vi "GDS1104B.vi"() -> ()   [LabVIEW 2014]
panel:
  out "number":u32
  out "read buffer 3":string
  out "read buffer 2":string
  out "before substring":string
  out "after substring":string
  out "Waveform Graph":cluster{dbl, dbl, dbl[]}(graph)
  out "Total Waveform Length":i32
  out "Waveform Start Time":dbl
  out "read buffer":string
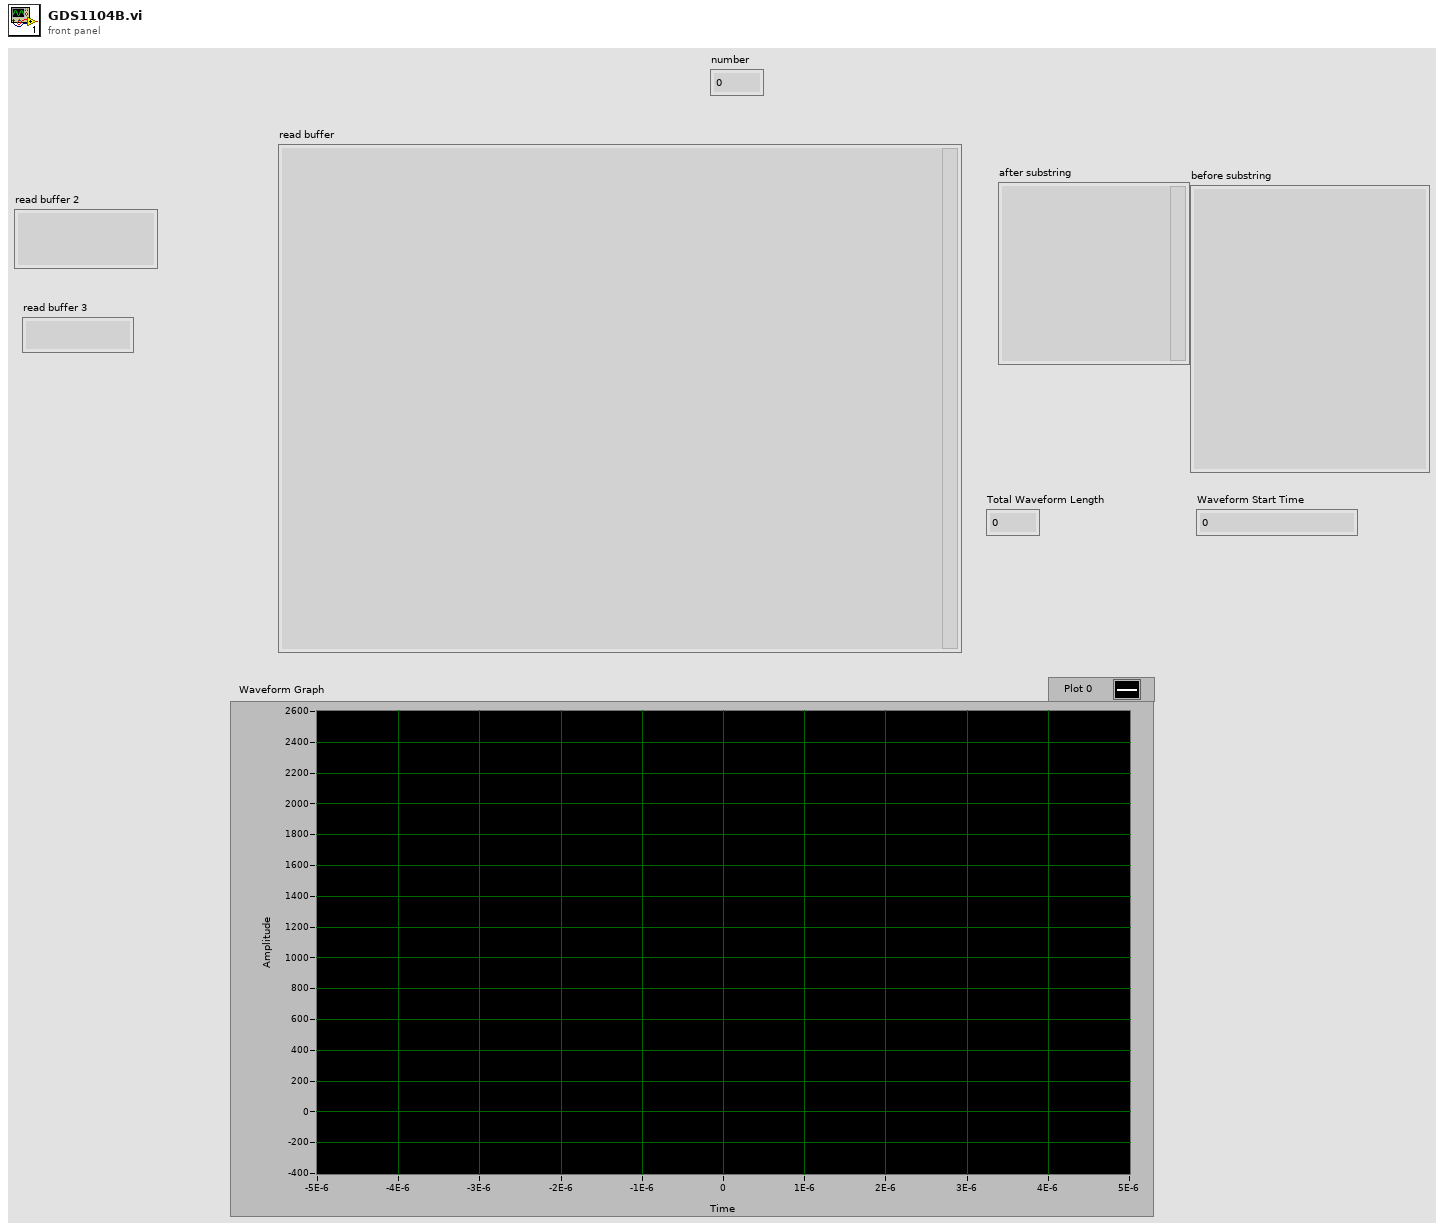
[diagram p1: front panel]
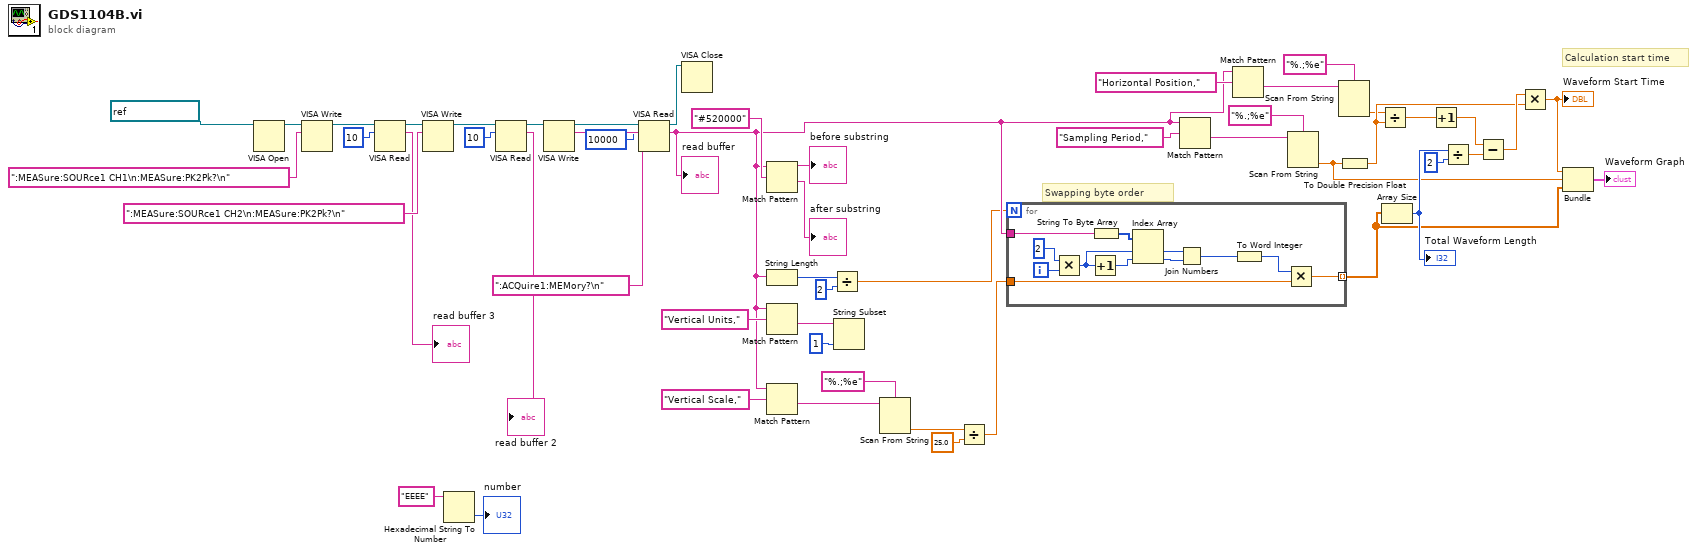
[diagram p0: block diagram]
diagram:
  # "Calculation start time"
  # "Swapping byte order"
  n1 = VISA Open(VISA resource name=refnum<visa-resource-name> "GDS1104B") -> (VISA resource name=w5:refnum<visa-resource-name>)  [unwired: 4 in, 1 out]
  n2 = VISA Write(VISA resource name=w5, write buffer=":MEASure:SOURce1 CH1\n:MEASure:PK2Pk?\n") -> (VISA resource name out=w11:refnum<visa-resource-name>)  [unwired: 1 in, 2 out]
  n3 = VISA Read(VISA resource name=w11, byte count=u32 10) -> (VISA resource name out=w9:refnum<visa-resource-name>, read buffer=→"read buffer 3":string)  [unwired: 1 in, 2 out]
  n4 = VISA Write(VISA resource name=w9, write buffer=":MEASure:SOURce1 CH2\n:MEASure:PK2Pk?\n") -> (VISA resource name out=w15:refnum<visa-resource-name>)  [unwired: 1 in, 2 out]
  n5 = Hexadecimal String To Number(string="EEEE") -> (number=→"number":u32)  [unwired: 2 in, 1 out]
  n6 = VISA Read(VISA resource name=w15, byte count=u32 10) -> (VISA resource name out=w6:refnum<visa-resource-name>, read buffer=→"read buffer 2":string)  [unwired: 1 in, 2 out]
  n7 = VISA Write(VISA resource name=w6, write buffer=":ACQuire1:MEMory?\n") -> (VISA resource name out=w4:refnum<visa-resource-name>)  [unwired: 1 in, 2 out]
  n8 = VISA Read(VISA resource name=w4, byte count=u32 10000) -> (VISA resource name out=w14:refnum<visa-resource-name>, read buffer=w23:string)  [unwired: 1 in, 2 out]
  "read buffer" <- w23
  n9 = VISA Close(VISA resource name=w14) -> ()  [unwired: 1 in, 1 out]
  n10 = Match Pattern(string=w23, regular expression="#520000") -> (before substring=→"before substring":string, after substring=→"after substring":string)  [unwired: 1 in, 2 out]
  n11 = String Length(string=w23) -> (length=w47:i32)
  n12 = Match Pattern(string=w23, regular expression="Vertical Units," ("y")) -> (after substring=w43:string)  [unwired: 1 in, 3 out]
  n13 = Match Pattern(string=w23, regular expression="Vertical Scale," ("y")) -> (after substring=w36:string)  [unwired: 1 in, 3 out]
  n14 = Divide(x=w47, y=2) -> (x/y=w22:dbl)
  n15 = String Subset(string=w43, length (rest)=1 ("length (rest)")) -> ()  [unwired: 1 in, 1 out]
  n16 = Scan From String(format string="%.;%e", input string=w36) -> (output 1=w35:dbl)  [unwired: 3 in, 3 out]
  n17 = Divide(x=w35, y=25.0) -> (x/y=w21:dbl)
  n18 = for {
    N: w22 -> [_]
    tunnel: [w58] -> w24 mode=indexing
    tunnel: w21 -> [w57]
    tunnel: w23 -> [w56]
    i -> [w60]
    n19 = Multiply(x=2 ("y"), y=w60) -> (x*y=w64:i32)
    n20 = Increment(x=w64) -> (x+1=w59:i32)
    n21 = String To Byte Array(string=w56) -> (unsigned byte array=w63:u8[])
    n22 = Index Array(array=w63, index #1=w64, index #2=w59) -> (element #1=w55:u8, element #2=w54:u8)
    n23 = Join Numbers(hi=w55, lo=w54) -> ((hi.lo)=w62:u16)
    n24 = To Word Integer(number=w62) -> (16bit integer=w53:i16)
    n25 = Multiply(x=w53, y=w57) -> (x*y=w58:dbl)
  }
  n26 = Match Pattern(string=w23, regular expression="Sampling Period," ("y")) -> (after substring=w34:string)  [unwired: 1 in, 3 out]
  n27 = Match Pattern(string=w23, regular expression="Horizontal Position," ("y")) -> (after substring=w40:string)  [unwired: 1 in, 3 out]
  n28 = Scan From String(format string="%.;%e", input string=w34) -> (output 1=w19:dbl)  [unwired: 3 in, 3 out]
  n29 = Scan From String(format string="%.;%e", input string=w40) -> (output 1=w20:dbl)  [unwired: 3 in, 3 out]
  n30 = To Double Precision Float(number=w19) -> (double precision float=w28:dbl)
  n31 = Divide(x=w20, y=w28) -> (x/y=w33:dbl)
  n32 = Array Size(array=w24) -> (size(s)=w27:i32)
  "Total Waveform Length" <- w27
  n33 = Increment(x=w33) -> (x+1=w32:dbl)
  n34 = Divide(x=w27, y=2) -> (x/y=w30:dbl)
  n35 = Subtract(x=w32, y=w30) -> (x-y=w29:dbl)
  n36 = Multiply(x=w29, y=w28) -> (x*y=w26:dbl)
  "Waveform Start Time" <- w26
  n37 = Bundle(w26, w19, w24) -> (→"Waveform Graph":cluster{dbl, dbl, dbl[]})  [unwired: 1 in]
